vi "from string 1.0.vi"(8 "error in (no error)":errorcluster, 10 "data":string, 11 "Formatter Config in":refnum<class "csv-formatter Config.lvclass">) -> (0 "error out":errorcluster, 3 "Formatter Config out":refnum<class "csv-formatter Config.lvclass">)   [LabVIEW 2015, in "csv-formatter Config.lvclass"]
uses:
  csv-formatter Config.lvclass
  Report Header Config.ctl
  Result Config.ctl
  csv-formatter Config.lvclass/csv-formatter Config.ctl
  <vilib>/NI/Configuration Framework/serializable configuration/NISE_CEF_serializable configuration.lvclass
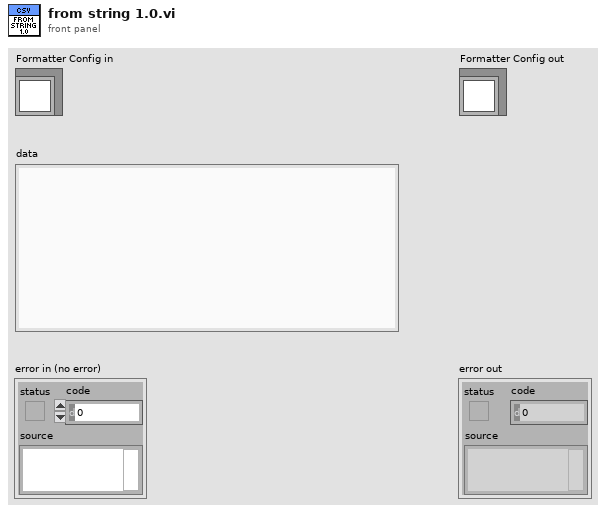
[diagram p1: front panel]
types:
  T1 = typedef "Result Config.ctl" = string[]
  T2 = typedef "Report Header Config.ctl" = string[][]
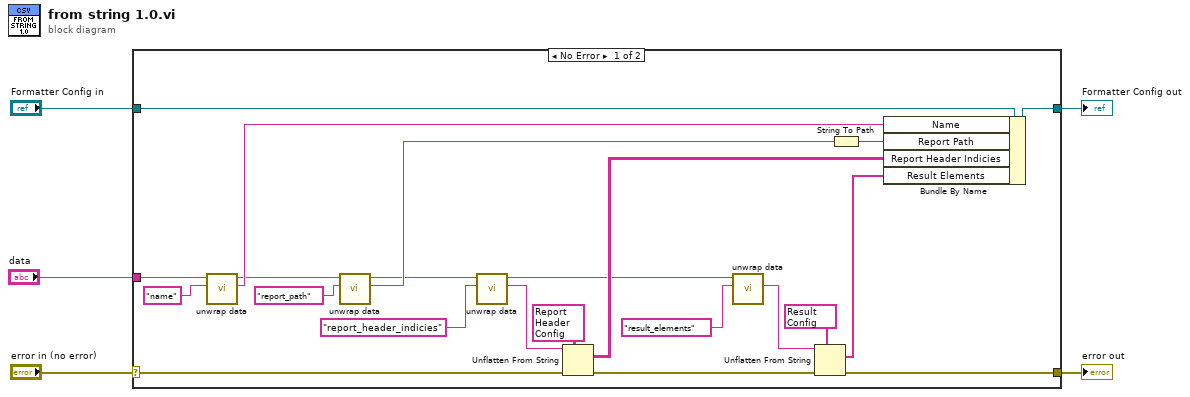
[diagram p0: block diagram]
diagram:
  n1 = case shown="No Error" "error in (no error)" {
    selector: "error in (no error)" -> [w16 w29]
    tunnel: [w9 w29] -> w4
    tunnel: [w26 w28] -> w2
    tunnel: "Formatter Config in" -> [w27 w28]
    tunnel: "data" -> [w25 _]
    frame No Error {
      n2 = call <vilib>:"unwrap data.vi"("identifier"="name", "data to unwrap"=w25) -> ("unwrapped data"=w23:string, "remaining string"=w22:string)  [unwired: 8 in]
      n3 = call <vilib>:"unwrap data.vi"("identifier"="report_path", "data to unwrap"=w22) -> ("unwrapped data"=w20:string, "remaining string"=w18:string)  [unwired: 8 in]
      n4 = call <vilib>:"unwrap data.vi"("identifier"="report_header_indicies", "data to unwrap"=w18) -> ("unwrapped data"=w15:string, "remaining string"=w8:string)  [unwired: 8 in]
      n5 = Unflatten From String(type=T2 [["UUT Result", "0", "0"], ["DUT Info", "0", "2"], ["DUT Serial Number", "0", "1"], ["Station Serial Number", "1", "0"], ["Station ID", "1", "1"]] ("Report Header Indicies"), binary string=w15, error in (no error)=w16) -> (value=w14:T2, error out=w12:errorcluster)  [unwired: 2 in, 1 out]
      n6 = call <vilib>:"unwrap data.vi"("identifier"="result_elements", "data to unwrap"=w8) -> ("unwrapped data"=w6:string)  [unwired: 8 in, 1 out]
      n7 = Unflatten From String(type=T1 ["Step Name", "Step Class", "Low Limit", "Measurement", "High Limit", "Comparison", "Duration"] ("Result Elements"), binary string=w6, error in (no error)=w12) -> (value=w10:T1, error out=w9:errorcluster)  [unwired: 2 in, 1 out]
      n8 = String To Path(string=w20) -> (path=w19:path)
      n9 = Bundle By Name(cluster=w27, "Name"=w23, "Report Path"=w19, "Report Header Indicies"=w14, "Result Elements"=w10) -> (w26:refnum<class "csv-formatter Config.lvclass">)
    }
    frame Error {
    }
  }
  "error out" <- w4
  "Formatter Config out" <- w2
